vi "设备配置界面.vi"() -> ()   [LabVIEW 2016, in "环境动力监测库.lvlib"]
uses:
  <vilib>/Utility/config.llb/NI_LVConfig.lvlib
panel:
  in  "设置默认配置":bool
  in  "一键恢复默认设置":bool
  in  "add3":bool
  in  "add2":bool
  in  "串口连接":enum16{"UPS监测", "空调监测"}(ring)
  in  "TCP连接":enum16{"UPS监测", "空调监测"}(ring)
  in  "设备列表":i32(listbox)
  in  "add":bool
  in  "IO连接":T1(ring)
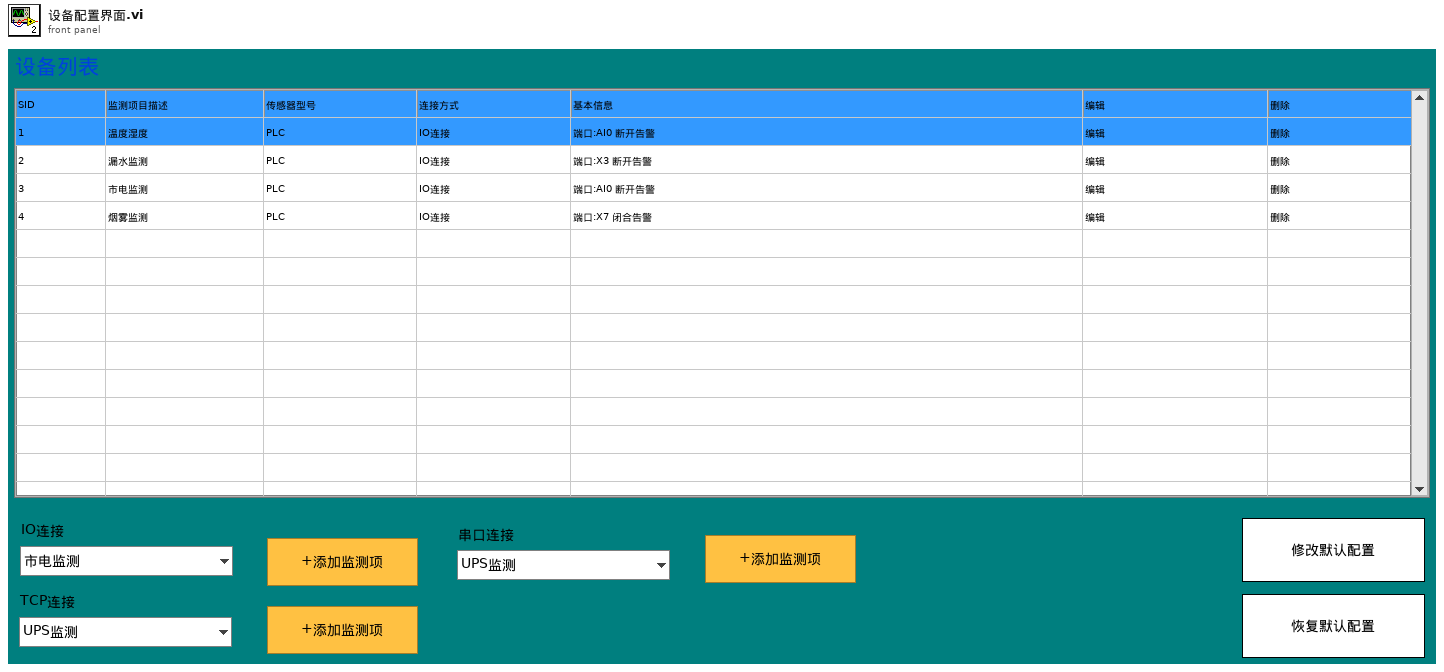
[diagram p1: front panel]
types:
  T1 = enum16{"市电监测", "用水量监测", "烟雾监测", "温度湿度", "振动监测", "红外入侵监测", "漏水监测", "门禁开关监测", "视频监测"}
  T2 = typedef "NI_LVConfig.lvlib/Config Data RefNum.ctl" = refnum<k1>
  T3 = cluster{"监测项描述:输出":string, "端口":string, "告警方式":string, "传感器型号":string}
  T4 = cluster{"监测项描述:输出":string, "IP":string, "port":string, "站号":string, "传感器型号":string, "波特率":string, "数据比特":string, "停止位":string, "奇偶校验":string}
  T5 = cluster{"监测项描述:输出":string, "端口":string, "站号":string, "传感器型号":string, "波特率":string, "停止位":string, "奇偶校验":string, "数据比特":string}
  T6 = typedef "LVPoint32TypeDef.ctl" = cluster{"Horizontal":i32, "Vertical":i32}
  T7 = typedef "LVRowAndColumnTypeDef.ctl" = cluster{"Row":i32, "Column":i32}
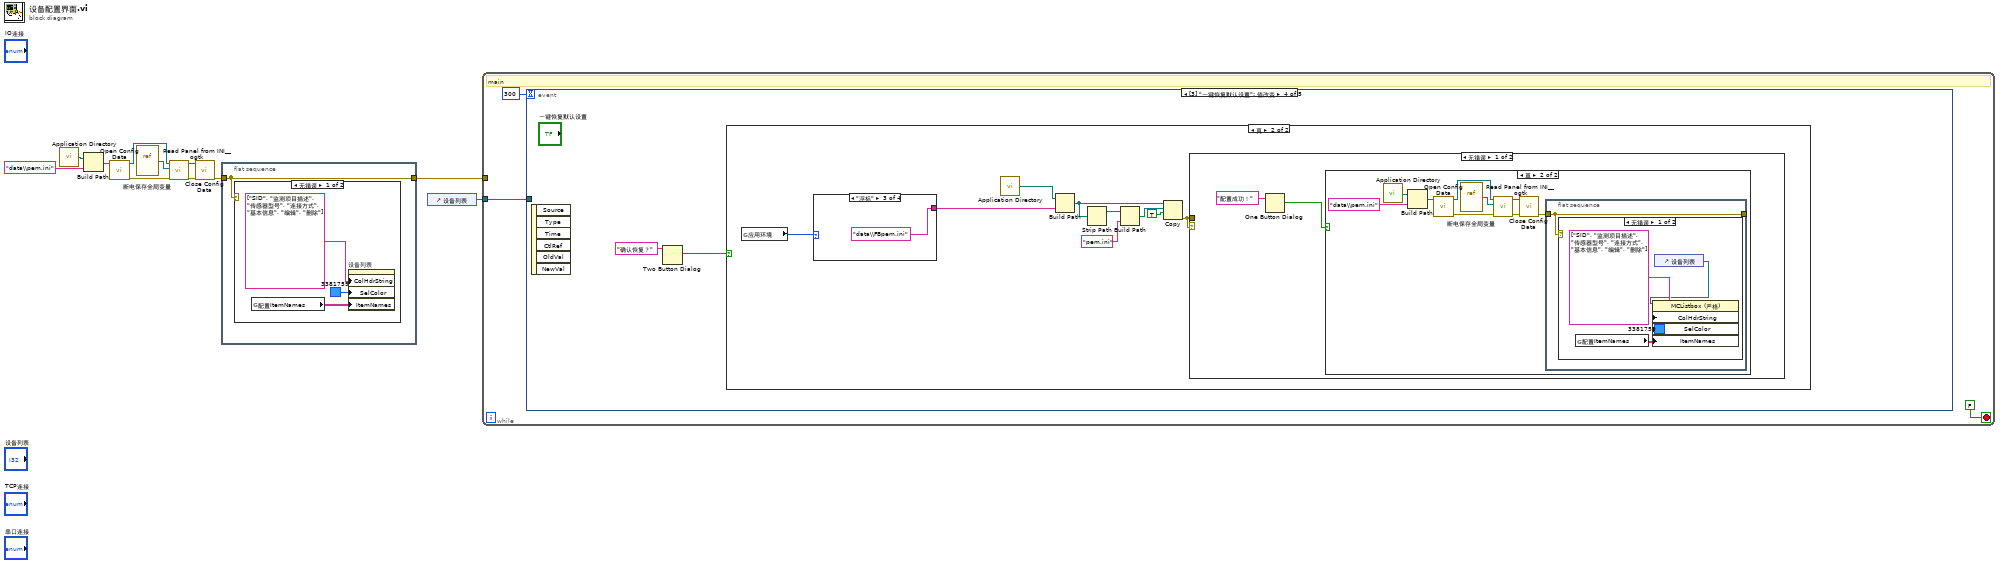
[diagram p0: block diagram]
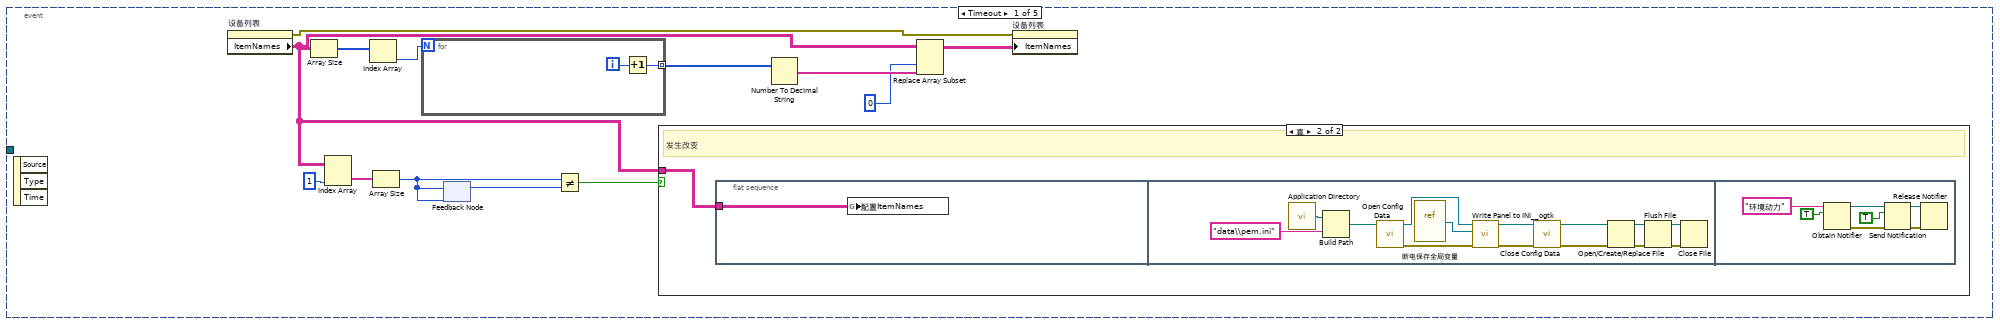
[diagram p3: hidden frame]
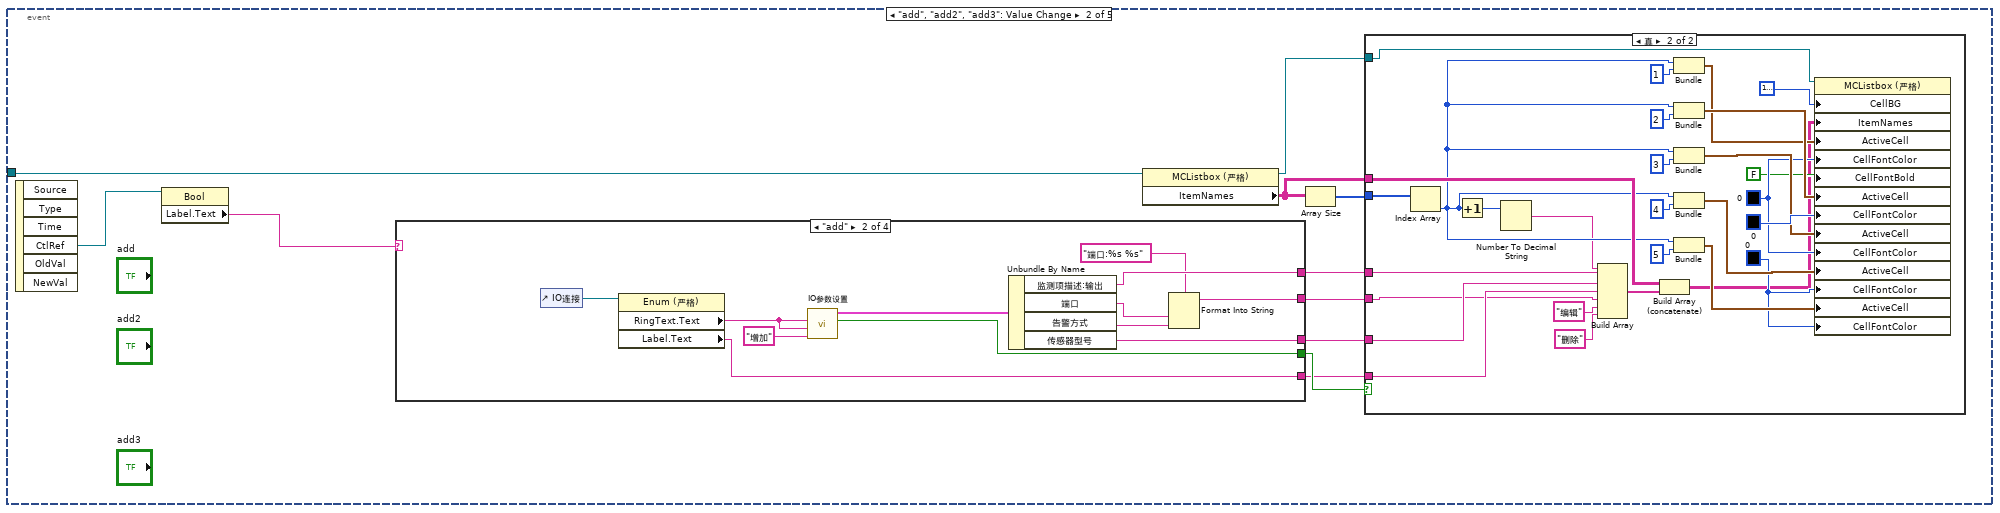
[diagram p5: hidden frame]
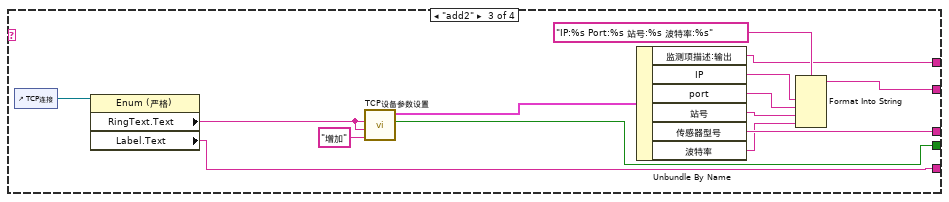
[diagram p7: hidden frame]
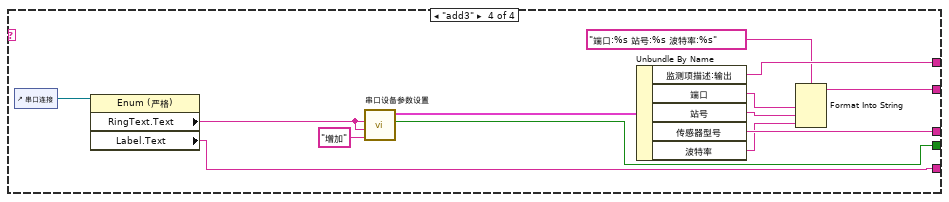
[diagram p8: hidden frame]
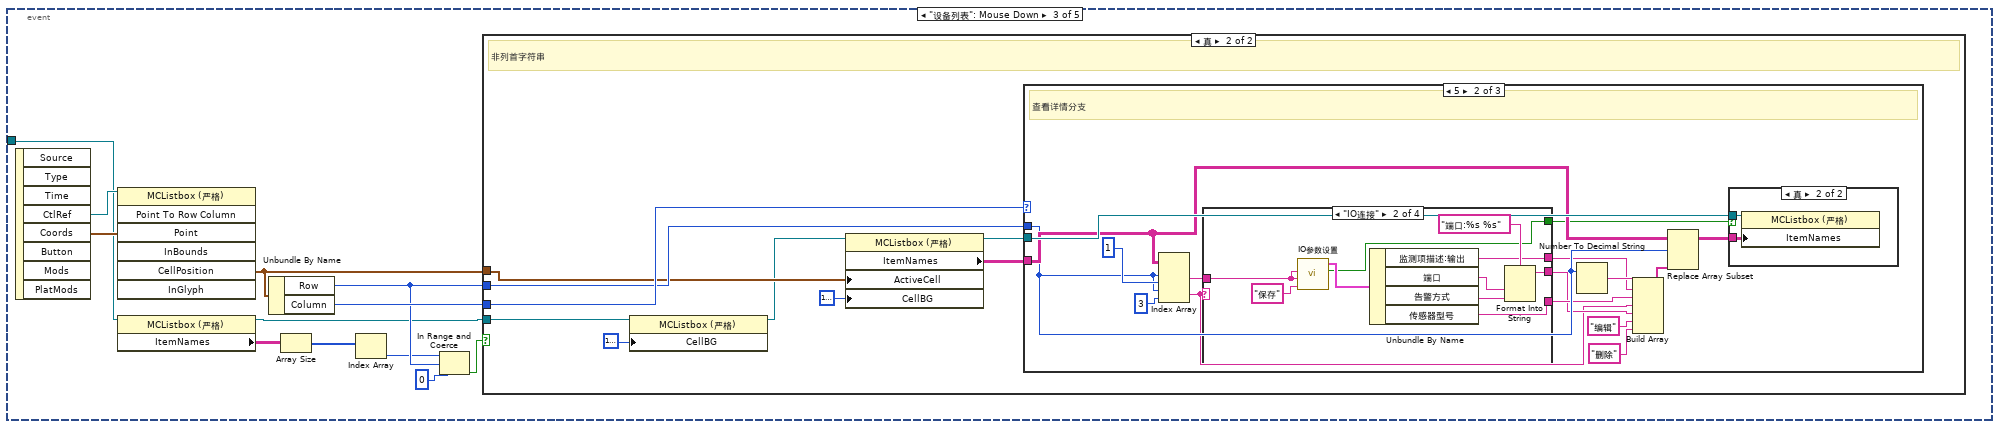
[diagram p10: hidden frame]
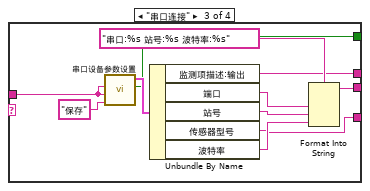
[diagram p15: hidden frame]
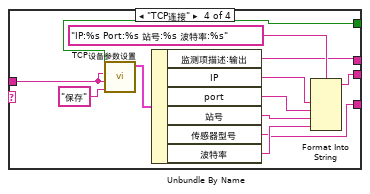
[diagram p16: hidden frame]
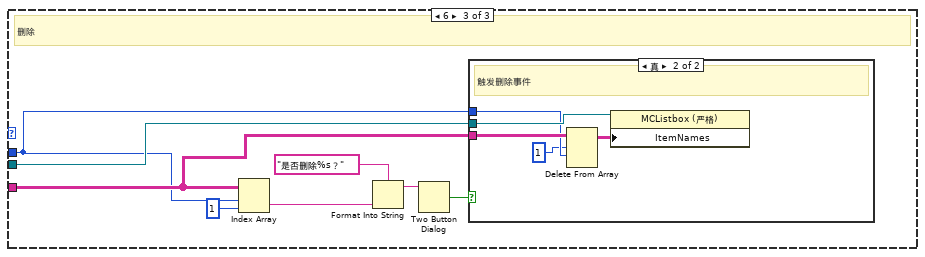
[diagram p17: hidden frame]
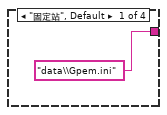
[diagram p20: hidden frame]
diagram:
  n1 = call <vilib>:"Application Directory.vi"() -> ("Application Directory"=w10:path)
  n2 = Build Path(base path=w10, name or relative path="data\\pem.ini" ("名称或相对路径")) -> (appended path=w8:path)
  n3 = call <vilib>:"Open Config Data.vi"("configuration file path"=w8) -> ("error out"=w4:errorcluster, "refnum"=w7:T2)  [unwired: 8 in, 1 out]
  n4 = vi-ref "断电保存全局变量.vi"() -> (w6:refnum<vi>)
  n5 = call <userlib>:"Read Panel from INI__ogtk.vi"("error in (no error)"=w4, "VI ref"=w6, "refnum"=w7) -> ("error out"=w3:errorcluster, "refnum out"=w5:T2)  [unwired: 7 in]
  n6 = call <vilib>:"Close Config Data.vi"("error in (no error)"=w3, "refnum"=w5) -> ("error out"=w2:errorcluster)  [unwired: 8 in, 1 out]
  n7 = flat-sequence {
    tunnel: w2 -> [w12]
    tunnel: [w12] -> w1
    frame #0 {
      n8 = case shown="无错误" w12 {
        frame No Error {
          n9 = global read "断电保存全局变量.vi" "配置ItemNames"() -> (w13:string[][])
          n10 = property on="设备列表" class="MCListbox (严格)"("ColHdrString"=string[] ["SID", "监测项目描述", "传感器型号", "连接方式", "基本信息", "编辑", "删除"] ("列首字符串[]"), "SelColor"=u32 3381759, "ItemNames"=w13) -> ()  [unwired: 2 in, 2 out]
        }
        frame Error {
        }
      }
    }
  }
  n11 = control-ref of="设备列表"() -> (w11:refnum<vi>)
  n12 = while {
    tunnel: w11 -> [w17]
    tunnel: w1 -> [_]
    stop <- FALSE stop-if-true
    # "main"
    n13 = event shown="[3] \"一键恢复默认设置\": 值改变" {
      selector: _ -> [_ _ _ _ _]
      dyn-events: _ -> [_ _ _ _ _]
      timeout: 300 -> [_ _ _ _ _]
      tunnel: w17 -> [_ w67 w141 _ _]
      event Timeout {
        n14 = event-data() -> ()  [unwired: 1 in, 3 out]
        n15 = property on="设备列表" class="MCListbox (严格)"() -> (error out=w30:errorcluster, "ItemNames"=w23:string[][])  [unwired: 2 in, 1 out]
        n16 = Array Size(array=w23) -> (size(s)=w31:i32[])
        n17 = Index Array(array=w23, index (col)=1 ("禁用的索引 (列)")) -> (element=w22:string[])  [unwired: 1 in]
        n18 = Index Array(array=w31) -> (element=w25:i32)  [unwired: 1 in]
        n19 = Array Size(array=w22) -> (size(s)=w20:i32)
        n20 = for {
          N: w25 -> [_]
          tunnel: [w55] -> w29 mode=indexing
          i -> [w56]
          n21 = Increment(x=w56) -> (x+1=w55:i32)
        }
        n22 = feedback-in #1(w20) -> ()
        n23 = feedback #1(w20) -> (w21:i32)
        n24 = Not Equal?(x=w20, y=w21) -> (x != y?=w19:bool)
        n25 = case shown="真" w19 {
          tunnel: w23 -> [_ w32]
          frame False {
          }
          frame True {
            # "发生改变"
            n26 = flat-sequence {
              tunnel: w32 -> [w33]
              frame #0 {
                n27 = global write "断电保存全局变量.vi" "配置ItemNames"(w33) -> ()
              }
              frame #1 {
                n28 = call <vilib>:"Application Directory.vi"() -> ("Application Directory"=w37:path)
                n29 = Build Path(base path=w37, name or relative path="data\\pem.ini" ("名称或相对路径")) -> (appended path=w36:path)
                n30 = call <vilib>:"Open Config Data.vi"("configuration file path"=w36) -> ("error out"=w35:errorcluster, "refnum"=w34:T2)  [unwired: 8 in, 1 out]
                n31 = vi-ref "断电保存全局变量.vi"() -> (w41:refnum<vi>)
                n32 = call <userlib>:"Write Panel to INI__ogtk.vi"("error in (no error)"=w35, "VI ref"=w41, "refnum"=w34) -> ("error out"=w40:errorcluster, "refnum out"=w39:T2)  [unwired: 7 in]
                n33 = call <vilib>:"Close Config Data.vi"("error in (no error)"=w40, "refnum"=w39) -> ("error out"=w47:errorcluster, "file path"=w46:path)  [unwired: 8 in]
                n34 = Open/Create/Replace File(file path (use dialog)=w46, error in=w47) -> (refnum out=w43:refnum<file>, error out=w42:errorcluster)  [unwired: 4 in, 1 out]
                n35 = Flush File(refnum=w43, error in=w42) -> (refnum out=w44:refnum<file>, error out=w45:errorcluster)
                n36 = Close File(refnum=w44, error in=w45) -> ()  [unwired: 2 out]
              }
              frame #2 {
                n37 = Obtain Notifier(name (unnamed)="环境动力" ("名称（未命名）"), notification data type=TRUE) -> (notifier out=w50:refnum<notifier>, error out=w51:errorcluster)  [unwired: 2 in, 1 out]
                n38 = Send Notification(notification=TRUE ("通知"), notifier=w50, error in (no error)=w51) -> (notifier out=w53:refnum<notifier>, error out=w54:errorcluster)
                n39 = Release Notifier(notifier=w53, error in (no error)=w54) -> ()  [unwired: 1 in, 3 out]
              }
            }
          }
        }
        n40 = Number To Decimal String(number=w29) -> (decimal integer string=w28:string[])  [unwired: 1 in]
        n41 = Replace Array Subset(array=w23, new element=w28, index (col)=0 ("禁用的索引 (列)")) -> (w26:string[][])  [unwired: 1 in]
        n42 = property on="设备列表" class="MCListbox (严格)"(error in=w30, "ItemNames"=w26) -> ()  [unwired: 1 in, 2 out]
      }
      event "add", "add2", "add3": Value Change {
        n43 = event-data() -> ("CtlRef"=w62:refnum<vi>)  [unwired: 1 in, 5 out]
        n44 = property class="Bool"(reference=w62) -> ("Label.Text"=w61:string)  [unwired: 1 in, 2 out]
        n45 = case shown="\"add\"" w61 {
          tunnel: [_ w79 w91 w105] -> w64
          tunnel: [_ w75 w89 w102] -> w60
          tunnel: [_ w73 w82 w100] -> w59
          tunnel: [_ w72 w87 w99] -> w58
          tunnel: [_ w68 w84 w94] -> w57
          frame "假", Default {
          }
          frame "add" {
            n46 = control-ref of="IO连接"() -> (w77:refnum<vi>)
            n47 = property class="Enum (严格)"(reference=w77) -> ("RingText.Text"=w76:string, "Label.Text"=w75:string)  [unwired: 1 in, 2 out]
            n48 = call "IO参数设置.vi"("布尔文本.文本"="增加", "section (optional)"=w76, "监测项描述"=w76) -> ("增加？"=w79:bool, "簇1输出"=w74:T3)  [unwired: 6 in, 1 out]
            n49 = Unbundle By Name(w74) -> ("监测项描述:输出"=w73:string, "端口"=w70:string, "告警方式"=w69:string, "传感器型号"=w72:string)
            n50 = Format Into String(format string="端口:%s %s" ("格式字符串"), w70, w69) -> (resulting string=w68:string)  [unwired: 2 in, 1 out]
          }
          frame "add2" {
            n51 = control-ref of="TCP连接"() -> (w93:refnum<vi>)
            n52 = property class="Enum (严格)"(reference=w93) -> ("RingText.Text"=w90:string, "Label.Text"=w89:string)  [unwired: 1 in, 2 out]
            n53 = call "TCP设备参数设置.vi"("布尔文本.文本"="增加" ("section (optional)"), "section (optional)"=w90, "监测项描述"=w90) -> ("布尔"=w91:bool, "输出簇"=w88:T4)  [unwired: 7 in]
            n54 = Unbundle By Name(w88) -> ("监测项描述:输出"=w82:string, "IP"=w81:string, "port"=w80:string, "站号"=w85:string, "传感器型号"=w87:string, "波特率"=w83:string)
            n55 = Format Into String(format string="IP:%s Port:%s 站号:%s 波特率:%s" ("格式字符串"), w81, w80, w85, w83) -> (resulting string=w84:string)  [unwired: 2 in, 1 out]
          }
          frame "add3" {
            n56 = control-ref of="串口连接"() -> (w103:refnum<vi>)
            n57 = property class="Enum (严格)"(reference=w103) -> ("RingText.Text"=w104:string, "Label.Text"=w102:string)  [unwired: 1 in, 2 out]
            n58 = call "串口设备参数设置.vi"("布尔文本.文本"="增加" ("section (optional)"), "section (optional)"=w104, "监测项描述"=w104) -> ("布尔"=w105:bool, "输出簇"=w101:T5)  [unwired: 7 in]
            n59 = Unbundle By Name(w101) -> ("监测项描述:输出"=w100:string, "端口"=w97:string, "站号"=w96:string, "传感器型号"=w99:string, "波特率"=w95:string)
            n60 = Format Into String(format string="端口:%s 站号:%s 波特率:%s" ("格式字符串"), w97, w96, w95) -> (resulting string=w94:string)  [unwired: 2 in, 1 out]
          }
        }
        n61 = property class="MCListbox (严格)"(reference=w67) -> (reference out=w65:refnum<vi>, "ItemNames"=w63:string[][])  [unwired: 1 in, 1 out]
        n62 = Array Size(array=w63) -> (size(s)=w66:i32[])
        n63 = case shown="真" w64 {
          tunnel: w63 -> [_ w134]
          tunnel: w66 -> [_ w133]
          tunnel: w65 -> [_ w131]
          tunnel: w60 -> [_ w113]
          tunnel: w59 -> [_ w110]
          tunnel: w58 -> [_ w109]
          tunnel: w57 -> [_ w108]
          frame False {
          }
          frame True {
            w114 = u32 0 ("颜色盒")
            w121 = u32 0 ("颜色盒")
            n64 = Index Array(array=w133) -> (element=w116:i32)  [unwired: 1 in]
            n65 = Increment(x=w116) -> (x+1=w132:i32)
            n66 = Number To Decimal String(number=w132) -> (decimal integer string=w111:string)  [unwired: 1 in]
            n67 = Build Array(w111, w110, w109, w113, w108, "编辑" ("元素"), "删除" ("元素")) -> (w135:string[])
            n68 = Build Array (concatenate)(w134, w135) -> (w112:string[][])
            n69 = Bundle(w116, "Column"=1) -> (w122:cluster{i32, "Column":i32})  [unwired: 1 in]
            n70 = Bundle(w116, "Column"=2) -> (w128:cluster{i32, "Column":i32})  [unwired: 1 in]
            n71 = Bundle(w116, "Column"=3) -> (w125:cluster{i32, "Column":i32})  [unwired: 1 in]
            n72 = Bundle(w116, "Column"=4) -> (w123:cluster{i32, "Column":i32})  [unwired: 1 in]
            n73 = Bundle(w116, "Column"=5) -> (w115:cluster{i32, "Column":i32})  [unwired: 1 in]
            n74 = property class="MCListbox (严格)"(reference=w131, "CellBG"=u32 16777216 ("颜色盒"), "ItemNames"=w112, "ActiveCell"=w122, "CellFontColor"=w121, "CellFontBold"=FALSE ("活动单元格:单元格字体:斜体"), "ActiveCell"=w128, "CellFontColor"=u32 0 ("颜色盒"), "ActiveCell"=w125, "CellFontColor"=w121, "ActiveCell"=w123, "CellFontColor"=w114, "ActiveCell"=w115, "CellFontColor"=w114) -> ()  [unwired: 1 in, 2 out]
          }
        }
      }
      event "设备列表": Mouse Down {
        n75 = event-data() -> ("CtlRef"=w147:refnum<vi>, "Coords"=w145:T6)  [unwired: 1 in, 6 out]
        n76 = invoke class="MCListbox (严格)" method="Point To Row Column"(reference=w147, "Point"=w145) -> ("CellPosition"=w144:T7)  [unwired: 5 in, 6 out]
        n77 = property class="MCListbox (严格)"(reference=w141) -> (reference out=w137:refnum<vi>, "ItemNames"=w140:string[][])  [unwired: 1 in, 1 out]
        n78 = Unbundle By Name(w144) -> ("Row"=w143:i32, "Column"=w146:i32)
        n79 = Array Size(array=w140) -> (size(s)=w139:i32[])
        n80 = Index Array(array=w139) -> (element=w138:i32)  [unwired: 1 in]
        n81 = In Range and Coerce(upper limit=w138, x=w143, lower limit=0 ("下限")) -> (In Range?=w136:bool)  [unwired: 1 out]
        n82 = case shown="真" w136 {
          tunnel: w146 -> [_ w155]
          tunnel: w143 -> [_ w154]
          tunnel: w144 -> [_ w152]
          tunnel: w137 -> [_ w149]
          frame False {
          }
          frame True {
            # "非列首字符串"
            n83 = property class="MCListbox (严格)"(reference=w149, "CellBG"=u32 16777216) -> (reference out=w150:refnum<vi>)  [unwired: 1 in, 1 out]
            n84 = property class="MCListbox (严格)"(reference=w150, "ActiveCell"=w152, "CellBG"=u32 16777216) -> (reference out=w153:refnum<vi>, "ItemNames"=w156:string[][])  [unwired: 1 in, 1 out]
            n85 = case shown="5" w155 {
              tunnel: w156 -> [_ w168 w215]
              tunnel: w154 -> [_ w163 w213]
              tunnel: w153 -> [_ w169 w214]
              frame 0, Default {
              }
              frame 5 {
                # "查看详情分支"
                n86 = Index Array(array=w168, index (row) #1=w163, index (col) #1=1 ("禁用的索引 (列)"), index (row) #2=w163, index (col) #2=3 ("禁用的索引 (列)")) -> (element #1=w171:string, element #2=w158:string)
                n87 = case shown="\"IO连接\"" w158 {
                  tunnel: w171 -> [_ w175 w185 w196]
                  tunnel: [_ w179 w189 w200] -> w161
                  tunnel: [_ w178 w187 w199] -> w159
                  tunnel: [_ w177 w188 w198] -> w160
                  tunnel: [_ w176 w186 w197] -> w157
                  frame "假", Default {
                  }
                  frame "IO连接" {
                    n88 = call "IO参数设置.vi"("布尔文本.文本"="保存", "section (optional)"=w175, "监测项描述"=w175) -> ("增加？"=w176:bool, "簇1输出"=w180:T3)  [unwired: 6 in, 1 out]
                    n89 = Unbundle By Name(w180) -> ("监测项描述:输出"=w179:string, "端口"=w182:string, "告警方式"=w181:string, "传感器型号"=w177:string)
                    n90 = Format Into String(format string="端口:%s %s" ("格式字符串"), w182, w181) -> (resulting string=w178:string)  [unwired: 2 in, 1 out]
                  }
                  frame "串口连接" {
                    n91 = call "串口设备参数设置.vi"("布尔文本.文本"="保存", "section (optional)"=w185, "监测项描述"=w185) -> ("布尔"=w186:bool, "输出簇"=w190:T5)  [unwired: 7 in]
                    n92 = Unbundle By Name(w190) -> ("监测项描述:输出"=w189:string, "端口"=w193:string, "站号"=w192:string, "传感器型号"=w188:string, "波特率"=w191:string)
                    n93 = Format Into String(format string="串口:%s 站号:%s 波特率:%s" ("格式字符串"), w193, w192, w191) -> (resulting string=w187:string)  [unwired: 2 in, 1 out]
                  }
                  frame "TCP连接" {
                    n94 = call "TCP设备参数设置.vi"("布尔文本.文本"="保存", "section (optional)"=w196, "监测项描述"=w196) -> ("布尔"=w197:bool, "输出簇"=w201:T4)  [unwired: 7 in]
                    n95 = Unbundle By Name(w201) -> ("监测项描述:输出"=w200:string, "IP"=w203:string, "port"=w202:string, "站号"=w205:string, "传感器型号"=w198:string, "波特率"=w204:string)
                    n96 = Format Into String(format string="IP:%s Port:%s 站号:%s 波特率:%s" ("格式字符串"), w203, w202, w205, w204) -> (resulting string=w199:string)  [unwired: 2 in, 1 out]
                  }
                }
                n97 = Number To Decimal String(number=w163) -> (decimal integer string=w162:string)  [unwired: 1 in]
                n98 = Build Array(w162, w161, w160, w158, w159, "编辑" ("元素"), "删除" ("元素")) -> (w164:string[])
                n99 = Replace Array Subset(array=w168, new element=w164, index (row)=w163) -> (w167:string[][])  [unwired: 1 in]
                n100 = case shown="真" w157 {
                  tunnel: w169 -> [_ w174]
                  tunnel: w167 -> [_ w173]
                  frame False {
                  }
                  frame True {
                    n101 = property class="MCListbox (严格)"(reference=w174, "ItemNames"=w173) -> ()  [unwired: 1 in, 2 out]
                  }
                }
              }
              frame 6 {
                # "删除"
                n102 = Index Array(array=w215, index (row)=w213, index (col)=1 ("禁用的索引 (列)")) -> (element=w209:string)
                n103 = Format Into String(format string="是否删除%s？" ("消息"), w209) -> (resulting string=w211:string)  [unwired: 2 in, 1 out]
                n104 = Two Button Dialog(message=w211) -> (T button?=w208:bool)  [unwired: 2 in]
                n105 = case shown="真" w208 {
                  tunnel: w214 -> [_ w220]
                  tunnel: w215 -> [_ w219]
                  tunnel: w213 -> [_ w218]
                  frame False {
                  }
                  frame True {
                    # "触发删除事件"
                    n106 = Delete From Array(array=w219, length=1 ("长度"), index (row)=w218) -> (array with subset deleted=w216:string[][])  [unwired: 1 in, 1 out]
                    n107 = property class="MCListbox (严格)"(reference=w220, "ItemNames"=w216) -> ()  [unwired: 1 in, 2 out]
                  }
                }
              }
            }
          }
        }
      }
      event "一键恢复默认设置": Value Change {
        n108 = event-data() -> ()  [unwired: 1 in, 6 out]
        n109 = Two Button Dialog(message="确认恢复？" ("消息")) -> (T button?=w221:bool)  [unwired: 2 in]
        n110 = case shown="真" w221 {
          frame False {
          }
          frame True {
            n111 = global read "外部交互全局变量.vi" "应用环境"() -> (w224:enum16{"固定站", "微站", "浮标", "浮船"})
            n112 = case shown="\"浮标\"" w224 {
              tunnel: ["data\\Gpem.ini" ("名称或相对路径") "data\\Vpem.ini" ("名称或相对路径") "data\\FBpem.ini" ("名称或相对路径") "data\\FCpem.ini" ("名称或相对路径")] -> w223
              frame "固定站", Default {
              }
              frame "微站" {
              }
              frame "浮标" {
              }
              frame "浮船" {
              }
            }
            n113 = call <vilib>:"Application Directory.vi"() -> ("Application Directory"=w231:path)
            n114 = Build Path(base path=w231, name or relative path=w223) -> (appended path=w225:path)
            n115 = Strip Path(path=w225) -> (stripped path=w229:path)  [unwired: 1 out]
            n116 = Build Path(base path=w229, name or relative path="pem.ini" ("名称或相对路径")) -> (appended path=w227:path)
            n117 = Copy(9:TRUE ("覆盖(F)"), 10:w227, 11:w225) -> (0:w226:errorcluster)  [unwired: 2 in, 2 out]
            n118 = case shown="无错误" w226 {
              tunnel: w226 -> [_ w253]
              frame No Error {
                n119 = One Button Dialog(message="配置成功！" ("消息")) -> (true=w236:bool)  [unwired: 1 in]
                n120 = case shown="真" w236 {
                  frame False {
                  }
                  frame True {
                    n121 = call <vilib>:"Application Directory.vi"() -> ("Application Directory"=w246:path)
                    n122 = Build Path(base path=w246, name or relative path="data\\pem.ini" ("名称或相对路径")) -> (appended path=w244:path)
                    n123 = call <vilib>:"Open Config Data.vi"("configuration file path"=w244) -> ("error out"=w240:errorcluster, "refnum"=w243:T2)  [unwired: 8 in, 1 out]
                    n124 = vi-ref "断电保存全局变量.vi"() -> (w242:refnum<vi>)
                    n125 = call <userlib>:"Read Panel from INI__ogtk.vi"("error in (no error)"=w240, "VI ref"=w242, "refnum"=w243) -> ("error out"=w239:errorcluster, "refnum out"=w241:T2)  [unwired: 7 in]
                    n126 = call <vilib>:"Close Config Data.vi"("error in (no error)"=w239, "refnum"=w241) -> ("error out"=w238:errorcluster)  [unwired: 8 in, 1 out]
                    n127 = flat-sequence {
                      tunnel: w238 -> [w247]
                      tunnel: [w247] -> _
                      frame #0 {
                        n128 = case shown="无错误" w247 {
                          frame No Error {
                            n129 = global read "断电保存全局变量.vi" "配置ItemNames"() -> (w249:string[][])
                            n130 = control-ref of="设备列表"() -> (w248:refnum<vi>)
                            n131 = property on="属性节点" class="MCListbox (严格)"(reference=w248, "ColHdrString"=string[] ["SID", "监测项目描述", "传感器型号", "连接方式", "基本信息", "编辑", "删除"] ("列首字符串[]"), "SelColor"=u32 3381759, "ItemNames"=w249) -> ()  [unwired: 1 in, 2 out]
                          }
                          frame Error {
                          }
                        }
                      }
                    }
                  }
                }
              }
              frame Error {
                n132 = Unbundle By Name(w253) -> ("code"=w252:i32)
                n133 = case shown="7" w252 {
                  frame 0, Default {
                  }
                  frame 7 {
                    n134 = One Button Dialog(message="找不到默认文件！" ("消息")) -> ()  [unwired: 1 in, 1 out]
                  }
                }
              }
            }
          }
        }
      }
      event "设置默认配置": Value Change {
        n135 = event-data() -> ()  [unwired: 1 in, 6 out]
        n136 = Two Button Dialog(message="确认将当前配置设置为默认配置？" ("消息")) -> (T button?=w255:bool)  [unwired: 2 in]
        n137 = case shown="真" w255 {
          frame False {
          }
          frame True {
            n138 = global read "外部交互全局变量.vi" "应用环境"() -> (w263:enum16{"固定站", "微站", "浮标", "浮船"})
            n139 = case shown="\"微站\"" w263 {
              tunnel: ["Gpem.ini" ("名称或相对路径") "Vpem.ini" ("名称或相对路径") "FBpem.ini" ("名称或相对路径") "FCpem.ini" ("名称或相对路径")] -> w265
              frame "固定站", Default {
              }
              frame "微站" {
              }
              frame "浮标" {
              }
              frame "浮船" {
              }
            }
            n140 = call <vilib>:"Application Directory.vi"() -> ("Application Directory"=w258:path)
            n141 = Build Path(base path=w258, name or relative path="data\\pem.ini" ("名称或相对路径")) -> (appended path=w262:path)
            n142 = Strip Path(path=w262) -> (stripped path=w260:path)  [unwired: 1 out]
            n143 = Build Path(base path=w260, name or relative path=w265) -> (appended path=w261:path)
            n144 = Copy(9:TRUE ("覆盖(F)"), 10:w261, 11:w262) -> (0:w257:errorcluster)  [unwired: 2 in, 2 out]
            n145 = case shown="无错误" w257 {
              frame No Error {
                n146 = One Button Dialog(message="配置成功！" ("消息")) -> ()  [unwired: 1 in, 1 out]
              }
              frame Error {
                n147 = One Button Dialog(message="配置失败！" ("消息")) -> ()  [unwired: 1 in, 1 out]
              }
            }
          }
        }
      }
    }
  }
